vi "Ballard - 1553 - Remote Terminal Sub Address.vi"(8 "error in (no error)":errorcluster, 11 "Node Ptr":T2 format="%.0x") -> (0 "error out":errorcluster)   [LabVIEW 2020, in "Ballard 1553 System Explorer.lvlib"]
uses:
  Ballard 1553 System Explorer.lvlib
  <vilib>/NI VeriStand/Custom Device API/Custom Device API.lvlib
  Shared/Controls and Global/Global.vi
  Shared/Ballard 1553 Shared.lvlib
  <vilib>/NI VeriStand/Custom Device API/Get Item Property (I32).vi
  <vilib>/NI VeriStand/Custom Device API/Get Item Property (U16).vi
  <vilib>/NI VeriStand/Custom Device API/Custom Device Item Ref.ctl
  SubVIs/Parse XML Ballard/Ballard_RT direction.ctl
panel:
  out "Direction":T1
  out "TA1":i8 caption="Sub-Address (SA 1)"
  in  "Header":cluster{"Section Name":string}={"Section Name"="Ballard - MIL-STD-1553 - Custom Device  - Remote Terminal Sub-Address"}
  in  "Description":string
  in  "Name":string
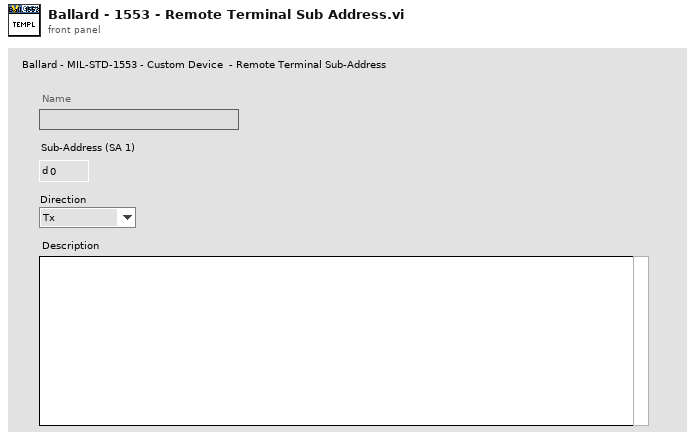
[diagram p1: front panel]
types:
  T1 = typedef "Ballard 1553 System Explorer.lvlib/Ballard_RT direction.ctl" = enum16{"Tx", "Rx"}
  T2 = typedef "Custom Device API.lvlib/Custom Device Item Ref.ctl" = u64
  T3 = typedef "Custom Device API.lvlib/Custom Device Item Info.ctl" = cluster{"Name":string, "Is Channel":bool, "GUID":string, "Is Waveform":bool}
  T4 = typedef "Custom Device API.lvlib/Custom Device Commands.ctl" = enum16{"Default", "Item renamed", "Shutdown", "Dynamic button pressed"}
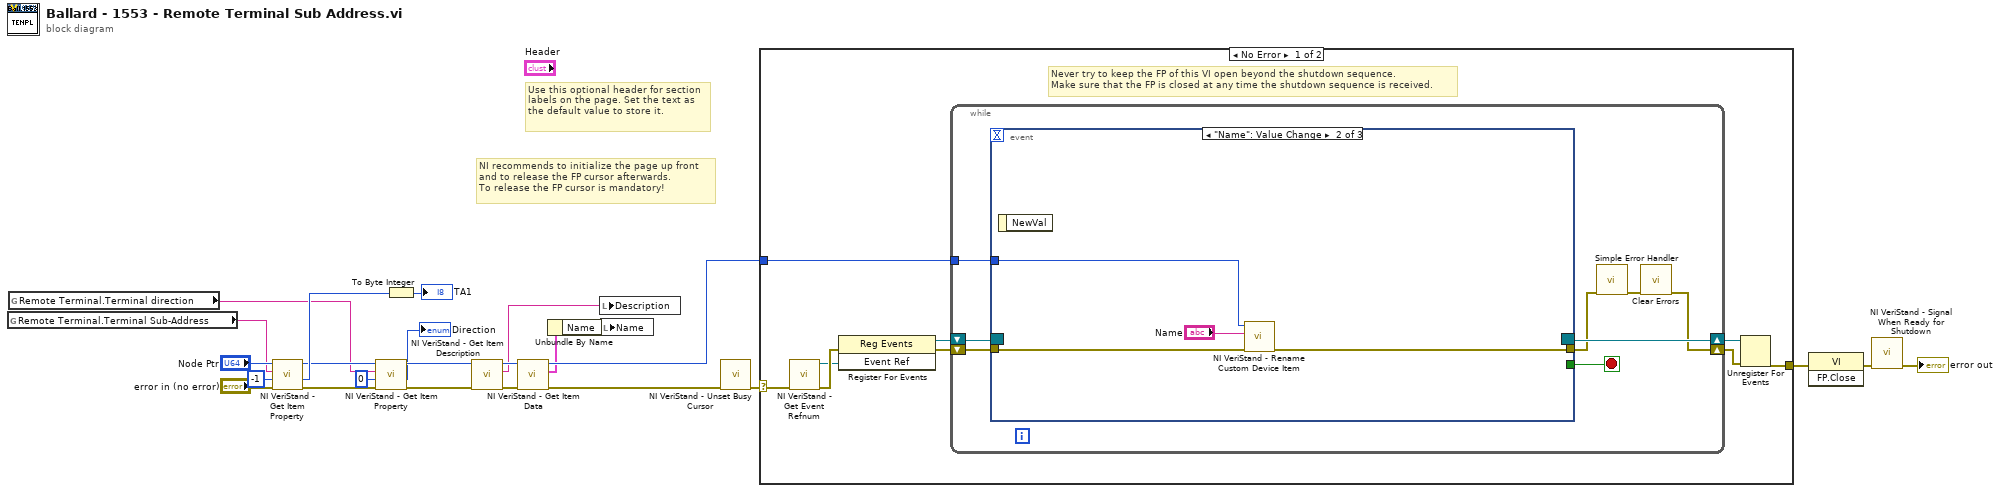
[diagram p0: block diagram]
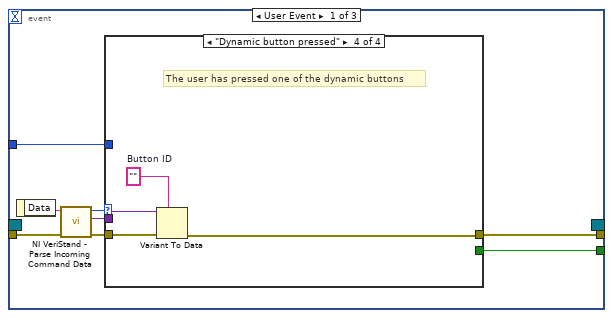
[diagram p2: hidden frame]
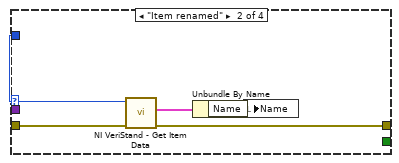
[diagram p4: hidden frame]
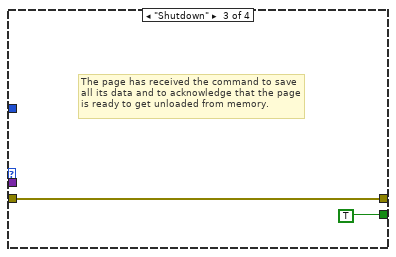
[diagram p5: hidden frame]
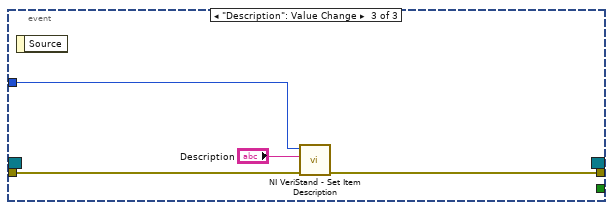
[diagram p6: hidden frame]
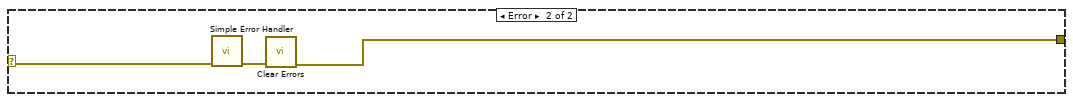
[diagram p7: hidden frame]
diagram:
  # "Use this optional header for section labels on the page. Set the text as the default value to store it."
  # "NI recommends to initialize the page up front\nand to release the FP cursor afterwards.\nTo release the FP cursor is mandatory!"
  n1 = global read "Global.vi" "Remote Terminal.Terminal Sub-Address"() -> (w1:string)
  n2 = global read "Global.vi" "Remote Terminal.Terminal direction"() -> (w2:string)
  n3 = call-poly <vilib>:"NI VeriStand - Get Item Property.vi"("error in (no error)"="error in (no error)", "Default Value"=-1, "Property Name"=w1, "Item Ref in"="Node Ptr") -> ("error out"=w7:errorcluster, "Value"=w11:i32, "Item Ref out"=w8:T2)  [unwired: 4 in, 1 out]
  n4 = call-poly <vilib>:"NI VeriStand - Get Item Property.vi"("error in (no error)"=w7, "Default Value"=u16 0, "Property Name"=w2, "Item Ref in"=w8) -> ("error out"=w5:errorcluster, "Value"=→"Direction":u16, "Item Ref out"=w6:T2)  [unwired: 4 in, 1 out]
  n5 = To Byte Integer(number=w11) -> (8bit integer=→"TA1":i8)
  n6 = call <vilib>:"NI VeriStand - Get Item Description.vi"("error in (no error)"=w5, "Item Ref in"=w6) -> ("error out"=w16:errorcluster, "Description"=w17:string, "Item Ref out"=w18:T2)  [unwired: 7 out]
  n7 = call <vilib>:"NI VeriStand - Get Item Data.vi"("error in (no error)"=w16, "Item Ref in"=w18) -> ("error out"=w21:errorcluster, "Item Info"=w15:T3, "Item Ref out"=w19:T2)  [unwired: 7 out]
  n8 = Unbundle By Name(w15) -> ("Name"=w14:string)
  n9 = local write "Description"(w17) -> ()
  n10 = local write "Name"(w14) -> ()
  n11 = call <vilib>:"NI VeriStand - Unset Busy Cursor.vi"("error in (no error)"=w21) -> ("error out"=w20:errorcluster)  [unwired: 10 out]
  n12 = case shown="No Error" w20 {
    selector: w20 -> [w25 w72]
    tunnel: [w30 w70] -> w24
    tunnel: w19 -> [w26 _]
    frame No Error {
      # "Never try to keep the FP of this VI open beyond the shutdown sequence.\nMake sure that the FP is closed at any time the shutdown sequence is received."
      n13 = call <vilib>:"NI VeriStand - Get Event Refnum.vi"("error in (no error)"=w25) -> ("error out"=w33:errorcluster, "Event Ref"=w29:refnum<user-event>)  [unwired: 9 out]
      n14 = register-events(error in=w33, w29) -> (reference out=w27:refnum<event-registration>, error out=w28:errorcluster)  [unwired: 1 in]
      n15 = while {
        tunnel: w26 -> [w37]
        shift-right: [w34] -> w31
        shift-left: w28 -> [w40]
        shift-right: [w41] -> w32
        shift-left: w27 -> [w39]
        stop <- w38 stop-if-true
        n16 = event shown="[1] \"Name\": Value Change" {
          selector: w39 -> [_ _ _]
          dyn-events: [_ _ _] -> w41
          timeout: _ -> [_ _ _]
          tunnel: w40 -> [w49 w65 w68]
          tunnel: [w45 _ _] -> w38
          tunnel: [w44 w64 w67] -> w36
          tunnel: w37 -> [w43 w63 w69]
          event User Event {
            n17 = event-data() -> ("Data"=w48:string)  [unwired: 1 out]
            n18 = call <vilib>:"NI VeriStand - Parse Incoming Command Data.vi"("error in (no error)"=w49, "Incoming data"=w48) -> ("error out"=w47:errorcluster, "Outgoing data"=w42:variant, "Action"=w46:T4)  [unwired: 7 out]
            n19 = case shown="\"Dynamic button pressed\"" w46 {
              tunnel: w47 -> [w50 w55 w56 w61]
              tunnel: [_ _ TRUE _] -> w45
              tunnel: [w50 w52 w56 w58] -> w44
              tunnel: w43 -> [_ w54 _ _]
              tunnel: w42 -> [_ _ _ w60]
              frame "Default", Default {
              }
              frame "Item renamed" {
                n20 = call <vilib>:"NI VeriStand - Get Item Data.vi"("error in (no error)"=w55, "Item Ref in"=w54) -> ("error out"=w52:errorcluster, "Item Info"=w53:T3)  [unwired: 8 out]
                n21 = Unbundle By Name(w53) -> ("Name"=w51:string)
                n22 = local write "Name"(w51) -> ()
              }
              frame "Shutdown" {
                # "The page has received the command to save all its data and to acknowledge that the page is ready to get unloaded from memory."
              }
              frame "Dynamic button pressed" {
                w59 = ""  # Button ID
                # "The user has pressed one of the dynamic buttons"
                n23 = Variant To Data(error in=w61, type=w59, Variant=w60) -> (error out=w58:errorcluster)  [unwired: 1 out]
              }
            }
          }
          event "Name": Value Change {
            n24 = event-data() -> ()  [unwired: 2 out]
            n25 = call <vilib>:"NI VeriStand - Rename Custom Device Item.vi"("error in (no error)"=w65, "New Name"="Name", "Item Ref in"=w63) -> ("error out"=w64:errorcluster)  [unwired: 1 in, 7 out]
          }
          event "Description": Value Change {
            n26 = event-data() -> ()  [unwired: 2 out]
            n27 = call <vilib>:"NI VeriStand - Set Item Description.vi"("error in (no error)"=w68, "Description"="Description", "Item Ref in"=w69) -> ("error out"=w67:errorcluster)  [unwired: 8 out]
          }
        }
        n28 = call <vilib>:"Simple Error Handler.vi"("error in (no error)"=w36) -> ("error out"=w35:errorcluster)  [unwired: 1 in, 7 out]
        n29 = call <vilib>:"Clear Errors.vi"("error in (no error)"=w35) -> ("error out"=w34:errorcluster)  [unwired: 1 in, 5 out]
      }
      n30 = Unregister For Events(event registration refnum=w32, error in=w31) -> (error out=w30:errorcluster)
    }
    frame Error {
      n31 = call <vilib>:"Simple Error Handler.vi"("error in (no error)"=w72) -> ("error out"=w71:errorcluster)  [unwired: 1 in, 7 out]
      n32 = call <vilib>:"Clear Errors.vi"("error in (no error)"=w71) -> ("error out"=w70:errorcluster)  [unwired: 1 in, 5 out]
    }
  }
  n33 = invoke class="VI" method="FP.Close"(error in=w24) -> (error out=w23:errorcluster)  [unwired: 2 in, 2 out]
  n34 = call <vilib>:"NI VeriStand - Signal When Ready for Shutdown.vi"("error in (no error)"=w23) -> ("error out"=→"error out":errorcluster)  [unwired: 10 out]
